vi "Write QO2 DVR.vi"(8 "error in (no error)":errorcluster, 10 "QO2 DVR":refnum<data-value>, 11 "Set Rel QO2 flow in":refnum<class "Set Rel QO2 flow.lvclass">) -> (0 "error out":errorcluster, 3 "Set Rel QO2 flow out":refnum<class "Set Rel QO2 flow.lvclass">)   [LabVIEW 2015, in "Set Rel QO2 flow.lvclass"]
uses:
  Set Rel QO2 flow.lvclass
  Set Rel QO2 flow.lvclass/Set Rel QO2 flow.ctl
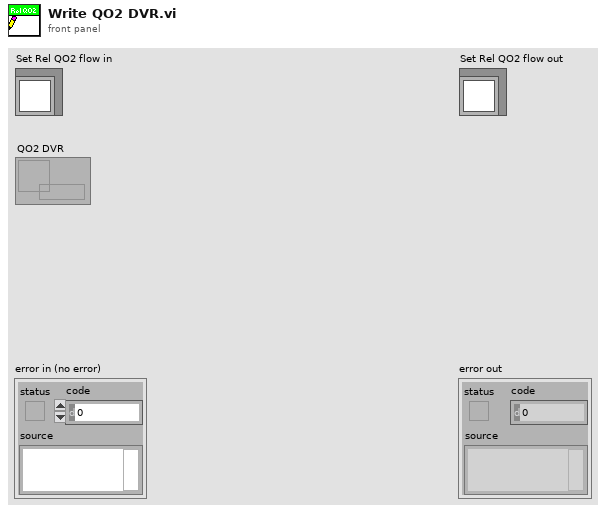
[diagram p1: front panel]
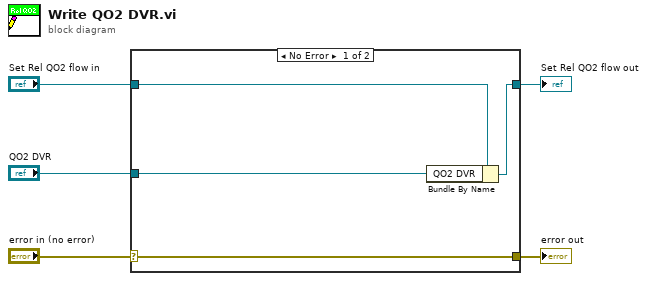
[diagram p0: block diagram]
diagram:
  n1 = case shown="No Error" "error in (no error)" {
    selector: "error in (no error)" -> [w9 w10]
    tunnel: [w9 w10] -> w4
    tunnel: [w7 w11] -> w2
    tunnel: "Set Rel QO2 flow in" -> [w8 w11]
    tunnel: "QO2 DVR" -> [w6 _]
    frame No Error {
      n2 = Bundle By Name(cluster=w8, "QO2 DVR"=w6) -> (w7:refnum<class "Set Rel QO2 flow.lvclass">)
    }
    frame Error {
    }
  }
  "error out" <- w4
  "Set Rel QO2 flow out" <- w2
